vi "Example Input.vi"() -> ()   [LabVIEW 2010]
uses:
  C:/tf/play/labview/Tinkerforge.dll
  Tinkerforge.dll
panel:
  out "value mask":bool[](array[boolean])
  in  "uid":string="cnq"
  in  "port":i32=4223
  in  "host":string="localhost"
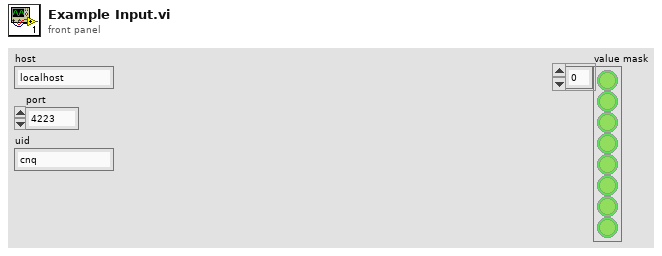
[diagram p1: front panel]
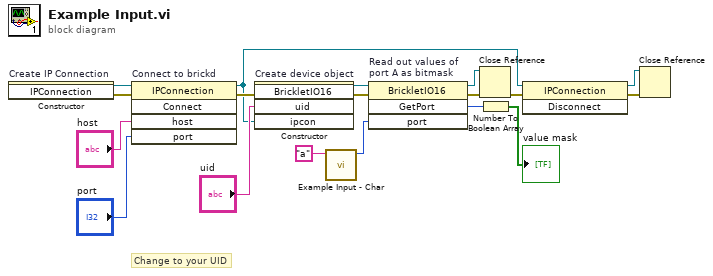
[diagram p0: block diagram]
diagram:
  # "Change to your UID"
  n1 = constructor on="Create IP Connection" class="IPConnection"() -> (reference out=w18:refnum<k24>, error out=w6:errorcluster)  [unwired: 3 in, 1 out]
  n2 = invoke on="Connect to brickd" class="IPConnection" method="Connect"(reference=w18, error in=w6, "host"="host", "port"="port") -> (reference out=w8:refnum<k24>, error out=w14:errorcluster)  [unwired: 1 in, 3 out]
  n3 = constructor on="Create device object" class="BrickletIO16"(error in=w14, "uid"="uid", "ipcon"=w8) -> (reference out=w13:refnum<k24>, error out=w3:errorcluster)  [unwired: 2 in, 3 out]
  n4 = call "Example Input - Char.vi"("string"="a") -> ("char"=w2:u16)  [unwired: 10 in]
  n5 = invoke on="Read out values of\nport A as bitmask" class="BrickletIO16" method="GetPort"(reference=w13, error in=w3, "port"=w2) -> (reference out=w11:refnum<k24>, error out=w12:errorcluster, "GetPort"=w4:u8)  [unwired: 1 in, 1 out]
  n6 = Close Reference(reference=w11, error in (no error)=w12) -> (error out=w10:errorcluster)
  n7 = Number To Boolean Array(number=w4) -> (Boolean array=→"value mask":bool[])
  n8 = invoke class="IPConnection" method="Disconnect"(reference=w8, error in=w10) -> (reference out=w7:refnum<k24>, error out=w9:errorcluster)  [unwired: 1 in, 1 out]
  n9 = Close Reference(reference=w7, error in (no error)=w9) -> ()  [unwired: 1 out]
